vi "Get Sections and Channels.vi"(8 "Error In":errorcluster, 11 "Custom Device Ref in":T1 format="%.0x") -> (0 "Error Out":errorcluster, 2 "Mux Data Array":T2[](array[typedef]), 3 "Custom Device Ref out":T1=18446744073709551615 format="%.0x")   [LabVIEW 2013, in "MUX Custom Device.lvlib"]
uses:
  MUX Custom Device.lvlib
  <vilib>/NI Veristand/Custom Device API/Custom Device Item Ref.ctl
  Mux Data.ctl
  Relay Channel Data.ctl
  Relay Data.ctl
  Switch.ctl
  MUX Global.vi
  <vilib>/NI Veristand/Custom Device API/Get Item Property (String).vi
  <vilib>/NI Veristand/Custom Device API/Custom Device API.lvlib
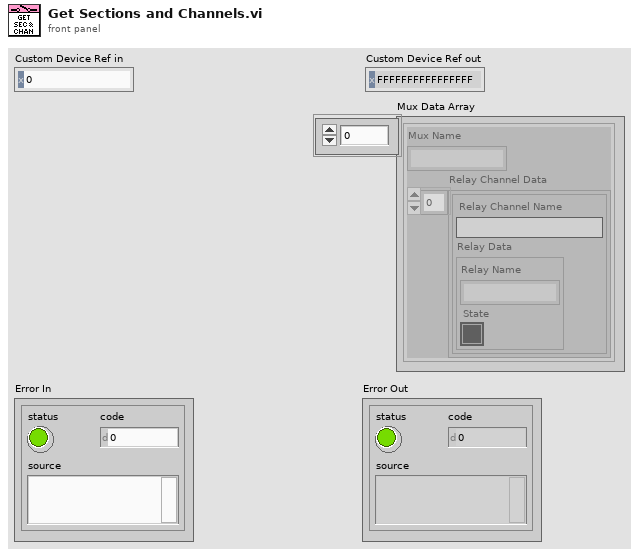
[diagram p1: front panel]
types:
  T1 = typedef "Custom Device API.lvlib/Custom Device Item Ref.ctl" = u64
  T2 = typedef "MUX Custom Device.lvlib/Mux Data.ctl" = cluster{"Mux Name":string, "Relay Channel Data":T3[]}
  T3 = typedef "MUX Custom Device.lvlib/Relay Channel Data.ctl" = cluster{"Relay Channel Name":string, "Relay Data":T4}
  T4 = typedef "MUX Custom Device.lvlib/Relay Data.ctl" = cluster{"Relay Name":string, "State":T5}
  T5 = typedef "MUX Custom Device.lvlib/Switch.ctl" = bool
  T6 = typedef "Custom Device API.lvlib/Custom Device Item Info.ctl" = cluster{"Name":string, "Is Channel":bool, "GUID":string, "Is Waveform":bool}
  T7 = typedef "Custom Device API.lvlib/Custom Device Channel.ctl" = cluster{"Type":T8, "Units":string, "Default Value":dbl, "Faultable":bool, "Scalable":bool}
  T8 = typedef "Custom Device API.lvlib/Custom Device Channel Type.ctl" = enum16{"Input", "Output"}
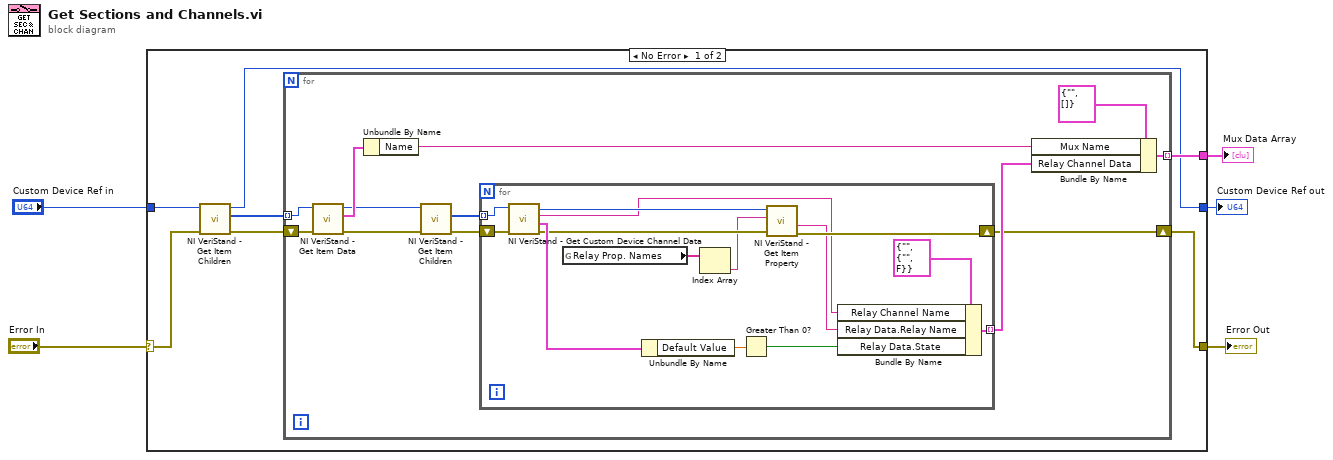
[diagram p0: block diagram]
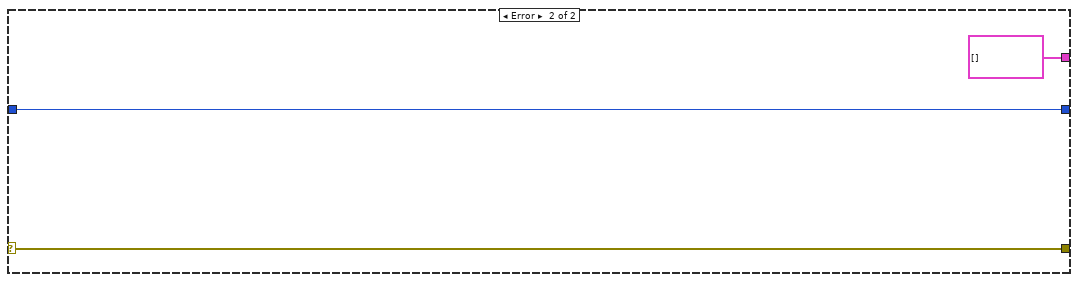
[diagram p2: hidden frame]
diagram:
  n1 = case shown="No Error" "Error In" {
    selector: "Error In" -> [w11 w41]
    tunnel: "Custom Device Ref in" -> [w12 w40]
    tunnel: [w6 w41] -> w3
    tunnel: [w7 w40] -> w2
    tunnel: [w10 T2[] [] ("Mux Data Array")] -> w1
    frame No Error {
      n2 = call <vilib>:"NI VeriStand - Get Item Children.vi"("error in (no error)"=w11, "Item Ref in"=w12) -> ("error out"=w9:errorcluster, "Child Refs"=w8:T1[], "Item Ref out"=w7:T1)  [unwired: 6 in, 1 out]
      n3 = for {
        tunnel: w8 -> [w23] mode=indexing
        tunnel: [w14] -> w10 mode=indexing
        shift-right: [w13] -> w6
        shift-left: w9 -> [w24]
        n4 = call <vilib>:"NI VeriStand - Get Item Data.vi"("error in (no error)"=w24, "Item Ref in"=w23) -> ("error out"=w20:errorcluster, "Item Info"=w22:T6, "Item Ref out"=w21:T1)  [unwired: 6 in, 1 out]
        n5 = Unbundle By Name(w22) -> ("Name"=w15:string)
        n6 = call <vilib>:"NI VeriStand - Get Item Children.vi"("error in (no error)"=w20, "Item Ref in"=w21) -> ("error out"=w18:errorcluster, "Child Refs"=w19:T1[])  [unwired: 6 in, 2 out]
        n7 = for {
          tunnel: w19 -> [w36] mode=indexing
          tunnel: [w33] -> w16 mode=indexing
          shift-right: [w27] -> w13
          shift-left: w18 -> [w37]
          n8 = call <vilib>:"NI VeriStand - Get Custom Device Channel Data.vi"("error in (no error)"=w37, "Channel Ref in"=w36) -> ("error out"=w31:errorcluster, "Channel"=w38:T7, "Channel Name"=w25:string, "Channel Ref out"=w30:T1)  [unwired: 4 in, 2 out]
          n9 = global read "MUX Global.vi" "Relay Prop. Names"() -> (w29:string[])
          n10 = Unbundle By Name(w38) -> ("Default Value"=w35:dbl)
          n11 = Index Array(array=w29) -> (element=w28:string)  [unwired: 1 in]
          n12 = Greater Than 0?(x=w35) -> (x > 0?=w34:bool)
          n13 = call-poly <vilib>:"NI VeriStand - Get Item Property.vi"("error in (no error)"=w31, "Property Name"=w28, "Item Ref in"=w30) -> ("error out"=w27:errorcluster, "Value"=w26:string)  [unwired: 5 in, 2 out]
          n14 = Bundle By Name(cluster=T3 {"Relay Channel Name"="", "Relay Data"={"Relay Name"="", "State"=FALSE}} ("Relay Channel Data"), "Relay Channel Name"=w25, "Relay Data.Relay Name"=w26, "Relay Data.State"=w34) -> (w33:T3)
        }
        n15 = Bundle By Name(cluster=T2 {"Mux Name"="", "Relay Channel Data"=[]} ("Mux Data"), "Mux Name"=w15, "Relay Channel Data"=w16) -> (w14:T2)
      }
    }
    frame Error {
    }
  }
  "Mux Data Array" <- w1
  "Error Out" <- w3
  "Custom Device Ref out" <- w2
